vi "claw work 1.vi"   [LabVIEW 2010, in "ClawBot.lvrbt"]
uses:
  ClawBot.lvrbt
  <vilib>/NXT/Block Support/NXT_InputPort.ctl
  <vilib>/NXT/Subs/MotorOutput.ctl
  <vilib>/NXT/Dual Mode Library/Sensors/Touch_Pressed.vi
  <vilib>/NXT/Dual Mode Library/Motors/ResetMotor.vi
  <vilib>/NXT/Dual Mode Library/Motors/MotorOn.vi
  <vilib>/NXT/Dual Mode Library/Motors/Rotation.vi
  <vilib>/NXT/Dual Mode Library/Motors/MotorBrake.vi
types:
  T1 = typedef "NXT_InputPort.ctl" = u8
  T2 = typedef "MotorOutput.ctl" = u8
  T3 = typedef "LVHSConnector.ctl" = cluster{"Hardware":string, "Flattened String":string}
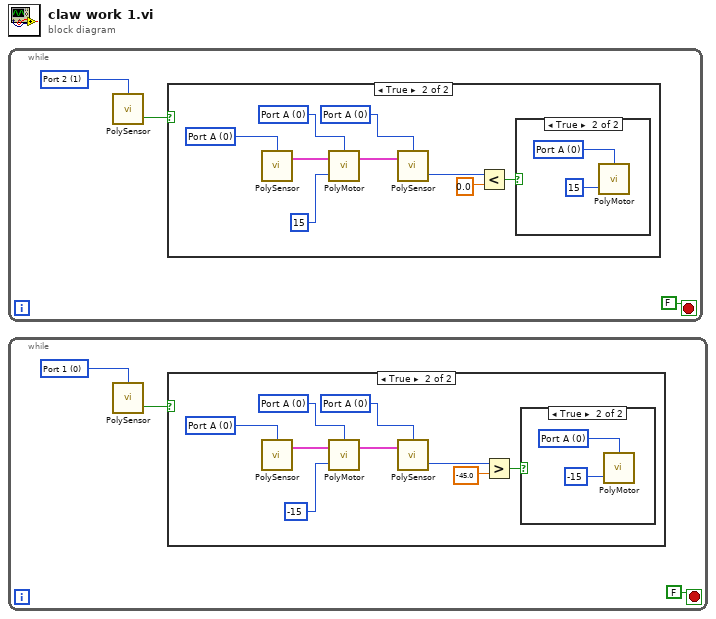
[diagram p0: block diagram]
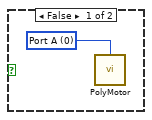
[diagram p3: hidden frame]
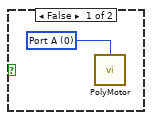
[diagram p5: hidden frame]
diagram:
  n1 = while {
    stop <- FALSE stop-if-true
    w2 = T1 1 items=["Port 1", "Port 2", "Port 3", "Port 4"] ("Port (Port 1)")
    n2 = call-poly <vilib>:"PolySensor.vi"("Port (Port 1)"=w2) -> ("Yes / No"=w3:bool)  [unwired: 2 in, 1 out]
    n3 = case shown="True" w3 {
      frame False {
      }
      frame True {
        w7 = T2 0 items=["Port A"=0, "Port B"=1, "Port C"=2, "Ports A & B"=4, "Ports A & C"=5, "Ports B & C"=6, "All Ports"=3] ("Port (All Ports)")
        w6 = u8 0 items=["Port A", "Port B", "Port C"] ("Port (Port A)")
        w4 = T2 0 items=["Port A"=0, "Port B"=1, "Port C"=2, "Ports A & B"=4, "Ports A & C"=5, "Ports B & C"=6, "All Ports"=3] ("Output Port (All Ports)")
        n4 = call-poly <vilib>:"PolySensor.vi"("Port (All Ports)"=w7) -> ("NXT"=w8:T3)  [unwired: 3 in]
        n5 = call-poly <vilib>:"PolyMotor.vi"("Power (75)"=15, "NXT"=w8, "Output Port (All Ports)"=w4) -> ("NXT"=w9:T3)  [unwired: 1 in]
        n6 = call-poly <vilib>:"PolySensor.vi"("NXT"=w9, "Port (Port A)"=w6) -> ("Angle of Rotation"=w10:i32)  [unwired: 1 in, 1 out]
        n7 = Less?(x=w10, y=0.0) -> (x < y?=w12:bool)
        n8 = case shown="True" w12 {
          frame False {
            w13 = T2 0 items=["Port A"=0, "Port B"=1, "Port C"=2, "Ports A & B"=4, "Ports A & C"=5, "Ports B & C"=6, "All Ports"=3] ("Output Port (All Ports)")
            n9 = call-poly <vilib>:"PolyMotor.vi"("Port (All Ports)"=w13) -> ()  [unwired: 3 in, 1 out]
          }
          frame True {
            w15 = T2 0 items=["Port A"=0, "Port B"=1, "Port C"=2, "Ports A & B"=4, "Ports A & C"=5, "Ports B & C"=6, "All Ports"=3] ("Output Port (All Ports)")
            n10 = call-poly <vilib>:"PolyMotor.vi"("Power (75)"=15, "Output Port (All Ports)"=w15) -> ()  [unwired: 2 in, 1 out]
          }
        }
      }
    }
  }
  n11 = while {
    stop <- FALSE stop-if-true
    w18 = T1 0 items=["Port 1", "Port 2", "Port 3", "Port 4"] ("Port (Port 1)")
    n12 = call-poly <vilib>:"PolySensor.vi"("Port (Port 1)"=w18) -> ("Yes / No"=w16:bool)  [unwired: 2 in, 1 out]
    n13 = case shown="True" w16 {
      frame False {
      }
      frame True {
        w24 = T2 0 items=["Port A"=0, "Port B"=1, "Port C"=2, "Ports A & B"=4, "Ports A & C"=5, "Ports B & C"=6, "All Ports"=3] ("Port (All Ports)")
        w25 = u8 0 items=["Port A", "Port B", "Port C"] ("Port (Port A)")
        w27 = T2 0 items=["Port A"=0, "Port B"=1, "Port C"=2, "Ports A & B"=4, "Ports A & C"=5, "Ports B & C"=6, "All Ports"=3] ("Output Port (All Ports)")
        n14 = call-poly <vilib>:"PolySensor.vi"("Port (All Ports)"=w24) -> ("NXT"=w23:T3)  [unwired: 3 in]
        n15 = call-poly <vilib>:"PolyMotor.vi"("Power (75)"=-15, "NXT"=w23, "Output Port (All Ports)"=w27) -> ("NXT"=w22:T3)  [unwired: 1 in]
        n16 = call-poly <vilib>:"PolySensor.vi"("NXT"=w22, "Port (Port A)"=w25) -> ("Angle of Rotation"=w20:i32)  [unwired: 1 in, 1 out]
        n17 = Greater?(x=w20, y=-45.0) -> (0:w19:bool)
        n18 = case shown="True" w19 {
          frame False {
            w28 = T2 0 items=["Port A"=0, "Port B"=1, "Port C"=2, "Ports A & B"=4, "Ports A & C"=5, "Ports B & C"=6, "All Ports"=3] ("Output Port (All Ports)")
            n19 = call-poly <vilib>:"PolyMotor.vi"("Port (All Ports)"=w28) -> ()  [unwired: 3 in, 1 out]
          }
          frame True {
            w30 = T2 0 items=["Port A"=0, "Port B"=1, "Port C"=2, "Ports A & B"=4, "Ports A & C"=5, "Ports B & C"=6, "All Ports"=3] ("Output Port (All Ports)")
            n20 = call-poly <vilib>:"PolyMotor.vi"("Power (75)"=-15, "Output Port (All Ports)"=w30) -> ()  [unwired: 2 in, 1 out]
          }
        }
      }
    }
  }
